vi "ItemSelected.vi"(8 "error in (no error)":errorcluster, 9 "Siblings":refnum<data-value>[](array[refnum]), 10 "MenuItem in":refnum<class "MGI_MenuItem.lvclass">, 11 "MGI_CheckmarkSelection in":refnum<class "MGI_CheckmarkSelection.lvclass">) -> (0 "error out":errorcluster, 2 "MenuItem out":refnum<class "MGI_MenuItem.lvclass">, 3 "MGI_CheckmarkSelection out":refnum<class "MGI_CheckmarkSelection.lvclass">)   [LabVIEW 2016, in "MGI_CheckmarkSelection.lvclass"]
doc: "Toggles the checkmark of the menu item.\n\nAuthored by Derek E. Trepanier\nsupport@mooregoodideas.com\nwww.mooregoodideas.com\n\nCopyright (c) 2012, Moore Good Ideas, Inc.\n\nAll rights reserved.\n\nRedistribution and use in source and binary forms, with or without modification, are permitted provided that the following conditions are met:\n\n * Redistributions of source code must retain the above copyright notice, this list of conditions and the following disclaimer.\n * Redistributions in binary form must reproduce the above copyright notice, this list of conditions and the following disclaimer in the documentation and/or other materials provided with the distribution.\n * Neither the name of Moore Good Ideas, Inc. nor the names of its contributors may be used to endorse or promote products derived from this software without specific prior written permission.\n\nTHIS SOFTWARE IS PROVIDED BY THE COPYRIGHT HOLDERS AND CONTRIBUTORS \"AS IS\" AND ANY EXPRESS OR IMPLIED WARRANTIES, INCLUDING, BUT NOT LIMITED TO, THE IMPLIED WARRANTIES OF MERCHANTABILITY AND FITNESS FOR A PARTICULAR PURPOSE ARE DISCLAIMED. IN NO EVENT SHALL THE COPYRIGHT OWNER OR CONTRIBUTORS BE LIABLE FOR ANY DIRECT, INDIRECT, INCIDENTAL, SPECIAL, EXEMPLARY, OR CONSEQUENTIAL DAMAGES (INCLUDING, BUT NOT LIMITED TO, PROCUREMENT OF SUBSTITUTE GOODS OR SERVICES; LOSS OF USE, DATA, OR PROFITS; OR BUSINESS INTERRUPTION) HOWEVER CAUSED AND ON ANY THEORY OF LIABILITY, WHETHER IN CONTRACT, STRICT LIABILITY, OR TORT (INCLUDING NEGLIGENCE OR OTHERWISE) ARISING IN ANY WAY OUT OF THE USE OF THIS SOFTWARE, EVEN IF ADVISED OF THE POSSIBILITY OF SUCH DAMAGE."
uses:
  <userlib>/_MGI/Menu Building/SelectionType/CheckmarkSelection/MGI_CheckmarkSelection.lvclass
  <userlib>/_MGI/Menu Building/MenuItem/MGI_MenuItem.lvclass
  <userlib>/_MGI/Menu Building/MenuItem/Read Checked.vi
  <userlib>/_MGI/Menu Building/MenuItem/Write Checked.vi
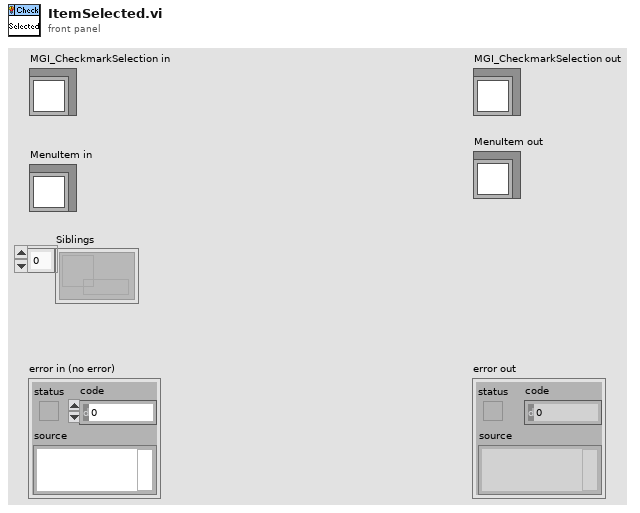
[diagram p1: front panel]
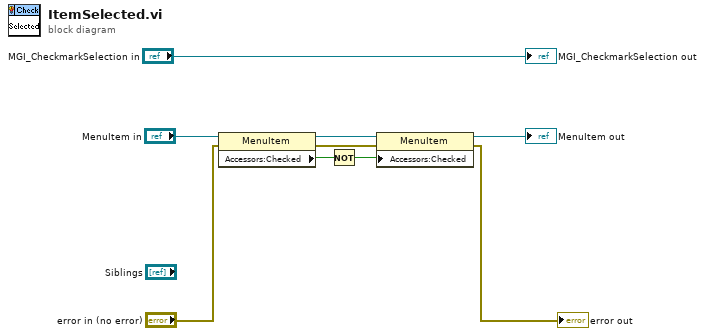
[diagram p0: block diagram]
diagram:
  n1 = property class="MenuItem"(reference="MenuItem in", error in="error in (no error)") -> (reference out=w7:refnum<class "MGI_MenuItem.lvclass">, error out=w2:errorcluster, "Accessors:Checked"=w5:bool)
  n2 = Not(x=w5) -> (.not. x?=w4:bool)
  n3 = property class="MenuItem"(reference=w7, error in=w2, "Accessors:Checked"=w4) -> (reference out=→"MenuItem out":refnum<class "MGI_MenuItem.lvclass">, error out=→"error out":errorcluster)
  "MGI_CheckmarkSelection out" <- "MGI_CheckmarkSelection in"
